vi "FindNumberOfTests.vi"(1 "Array":string[][](array[string])) -> (0 "Numeric":i32)   [LabVIEW 2010]
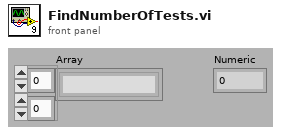
[diagram p1: front panel]
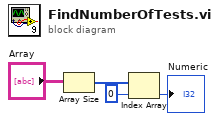
[diagram p0: block diagram]
diagram:
  n1 = Array Size(array="Array") -> (size(s)=w2:i32[])
  n2 = Index Array(array=w2, index=0) -> (element=→"Numeric":i32)
